vi "New Error Pointer.vi"(8 "error in (no error)":errorcluster, 11 "Thread in":refnum<class "Thread.lvclass">) -> (0 "error out":errorcluster, 3 "Thread out":refnum<class "Thread.lvclass">)   [LabVIEW 2017, in "DSF Core.lvlib" / "Thread.lvclass"]
uses:
  Thread.lvclass
  Thread.lvclass/Thread.ctl
  Pointers/Error/Error Pointer.lvclass
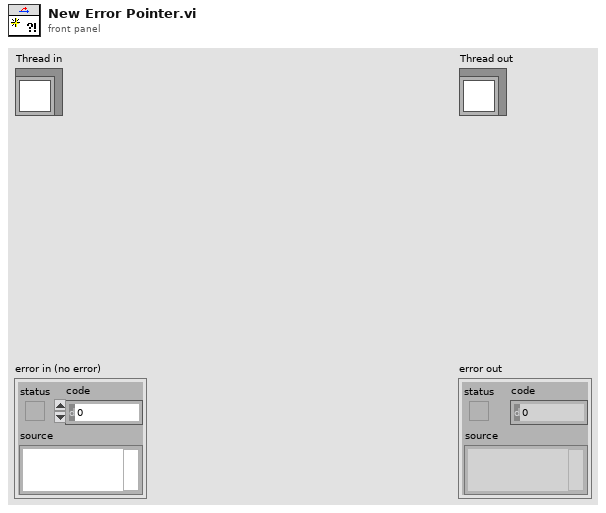
[diagram p1: front panel]
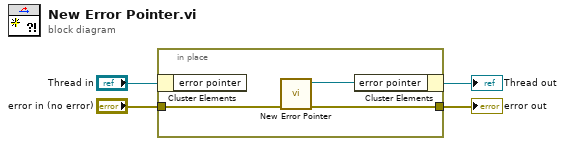
[diagram p0: block diagram]
diagram:
  n1 = in-place {
    in-place-border: [w6] -> w3
    in-place-border: "error in (no error)" -> [w5]
    n2 = in-place-cluster #1("Thread in") -> ()  [unwired: 1 out]
    n3 = call "New Error Pointer.vi"("error in (no error)"=w5) -> ("error out"=w6:errorcluster, "Error Pointer out"=w7:refnum<class "Error Pointer.lvclass">)  [unwired: 9 in]
    n4 = in-place-cluster #1("error pointer"=w7) -> (→"Thread out":refnum<class "Thread.lvclass">)
  }
  "error out" <- w3
